vi "Actor Core.vi"(8 "error in":errorcluster, 11 "SignalProcessing in":refnum<class "SignalProcessing.lvclass">) -> (0 "error out":errorcluster, 3 "Actor out":refnum<class "Actor.lvclass">)   [LabVIEW 2019, in "SignalProcessing.lvlib" / "SignalProcessing.lvclass"]
doc: "(<B>Filename</B>: Actor Framework.lvlib:Actor.lvclass:Actor Core.vi)\n\nReceives messages to the actor, reacts to them, and initiates any error handling that may shut the actor down.\n\nDescendant classes may override this VI to append parallel tasks for the actor to complete while it handles messages. Overrides use the Call Parent Method node."
uses:
  SignalProcessing.lvclass
  C:/Program Files (x86)/National Instruments/LabVIEW 2019/vi.lib/ActorFramework/Actor/Actor.lvclass
  <vilib>/ActorFramework/Actor/Actor.lvclass
  SignalProcessing.lvclass/SignalProcessing.ctl
  <vilib>/ActorFramework/Actor/Actor.lvclass/Actor.ctl
  <vilib>/ActorFramework/Message Enqueuer/Message Enqueuer.lvclass/Message Enqueuer.ctl
  LunchTest.lvclass
  C:/Program Files (x86)/National Instruments/LabVIEW 2019/vi.lib/NI/Event Source Actor/Event Source/Event/Event.lvclass
  <vilib>/NI/Event Source Actor/Event Source/Event/Event.lvclass/Event.ctl
  <vilib>/NI/Event Source Actor/Event Source/Event Source Messages/Generate Event Msg/Generate Event Msg.lvclass/Generate Event Msg.ctl
  Exit.lvclass
  <vilib>/ActorFramework/Message Enqueuer/Init from Existing Queue.vi
  <vilib>/ActorFramework/Message Enqueuer/Enqueue.vi
  <vilib>/NI/Event Source Actor/Event Source/Event Source Messages/Generate Event Msg/Generate Event Msg.lvclass
  C:/Program Files (x86)/National Instruments/LabVIEW 2019/vi.lib/ActorFramework/Message/Message.lvclass
  SignalProcessing Global.vi
  <vilib>/ActorFramework/Message Priority Queue/Priority Enqueue.vi
  <vilib>/NI/Event Source Actor/Event Source/Event Source/Event Source.lvclass
  <vilib>/ActorFramework/Message Enqueuer/Message Enqueuer.lvclass
  <vilib>/NI/Event Source Actor/Event Source/Event/Event.lvclass
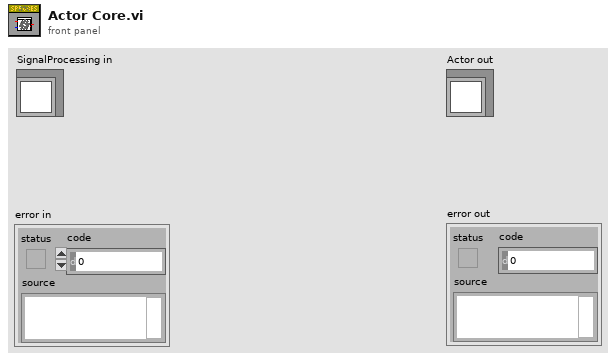
[diagram p1: front panel]
types:
  T1 = enum32{"Invalid", "Standard", "Closed", "Hidden", "Minimized", "Maximized"}
  T2 = enum32{"invalid app kind", "Development System", "Run Time System", "Student Edition", "Embedded LabVIEW", "Evaluation", "Custom"}
  T3 = cluster{"Core":cluster{"Current VI Reference":refnum<vi>, "Close Panel on Exit?":bool}, "Your Boolean data":bool, "Your string data":string}
  T4 = cluster{"Current VI Reference":refnum<vi>, "Close Panel on Exit?":bool}
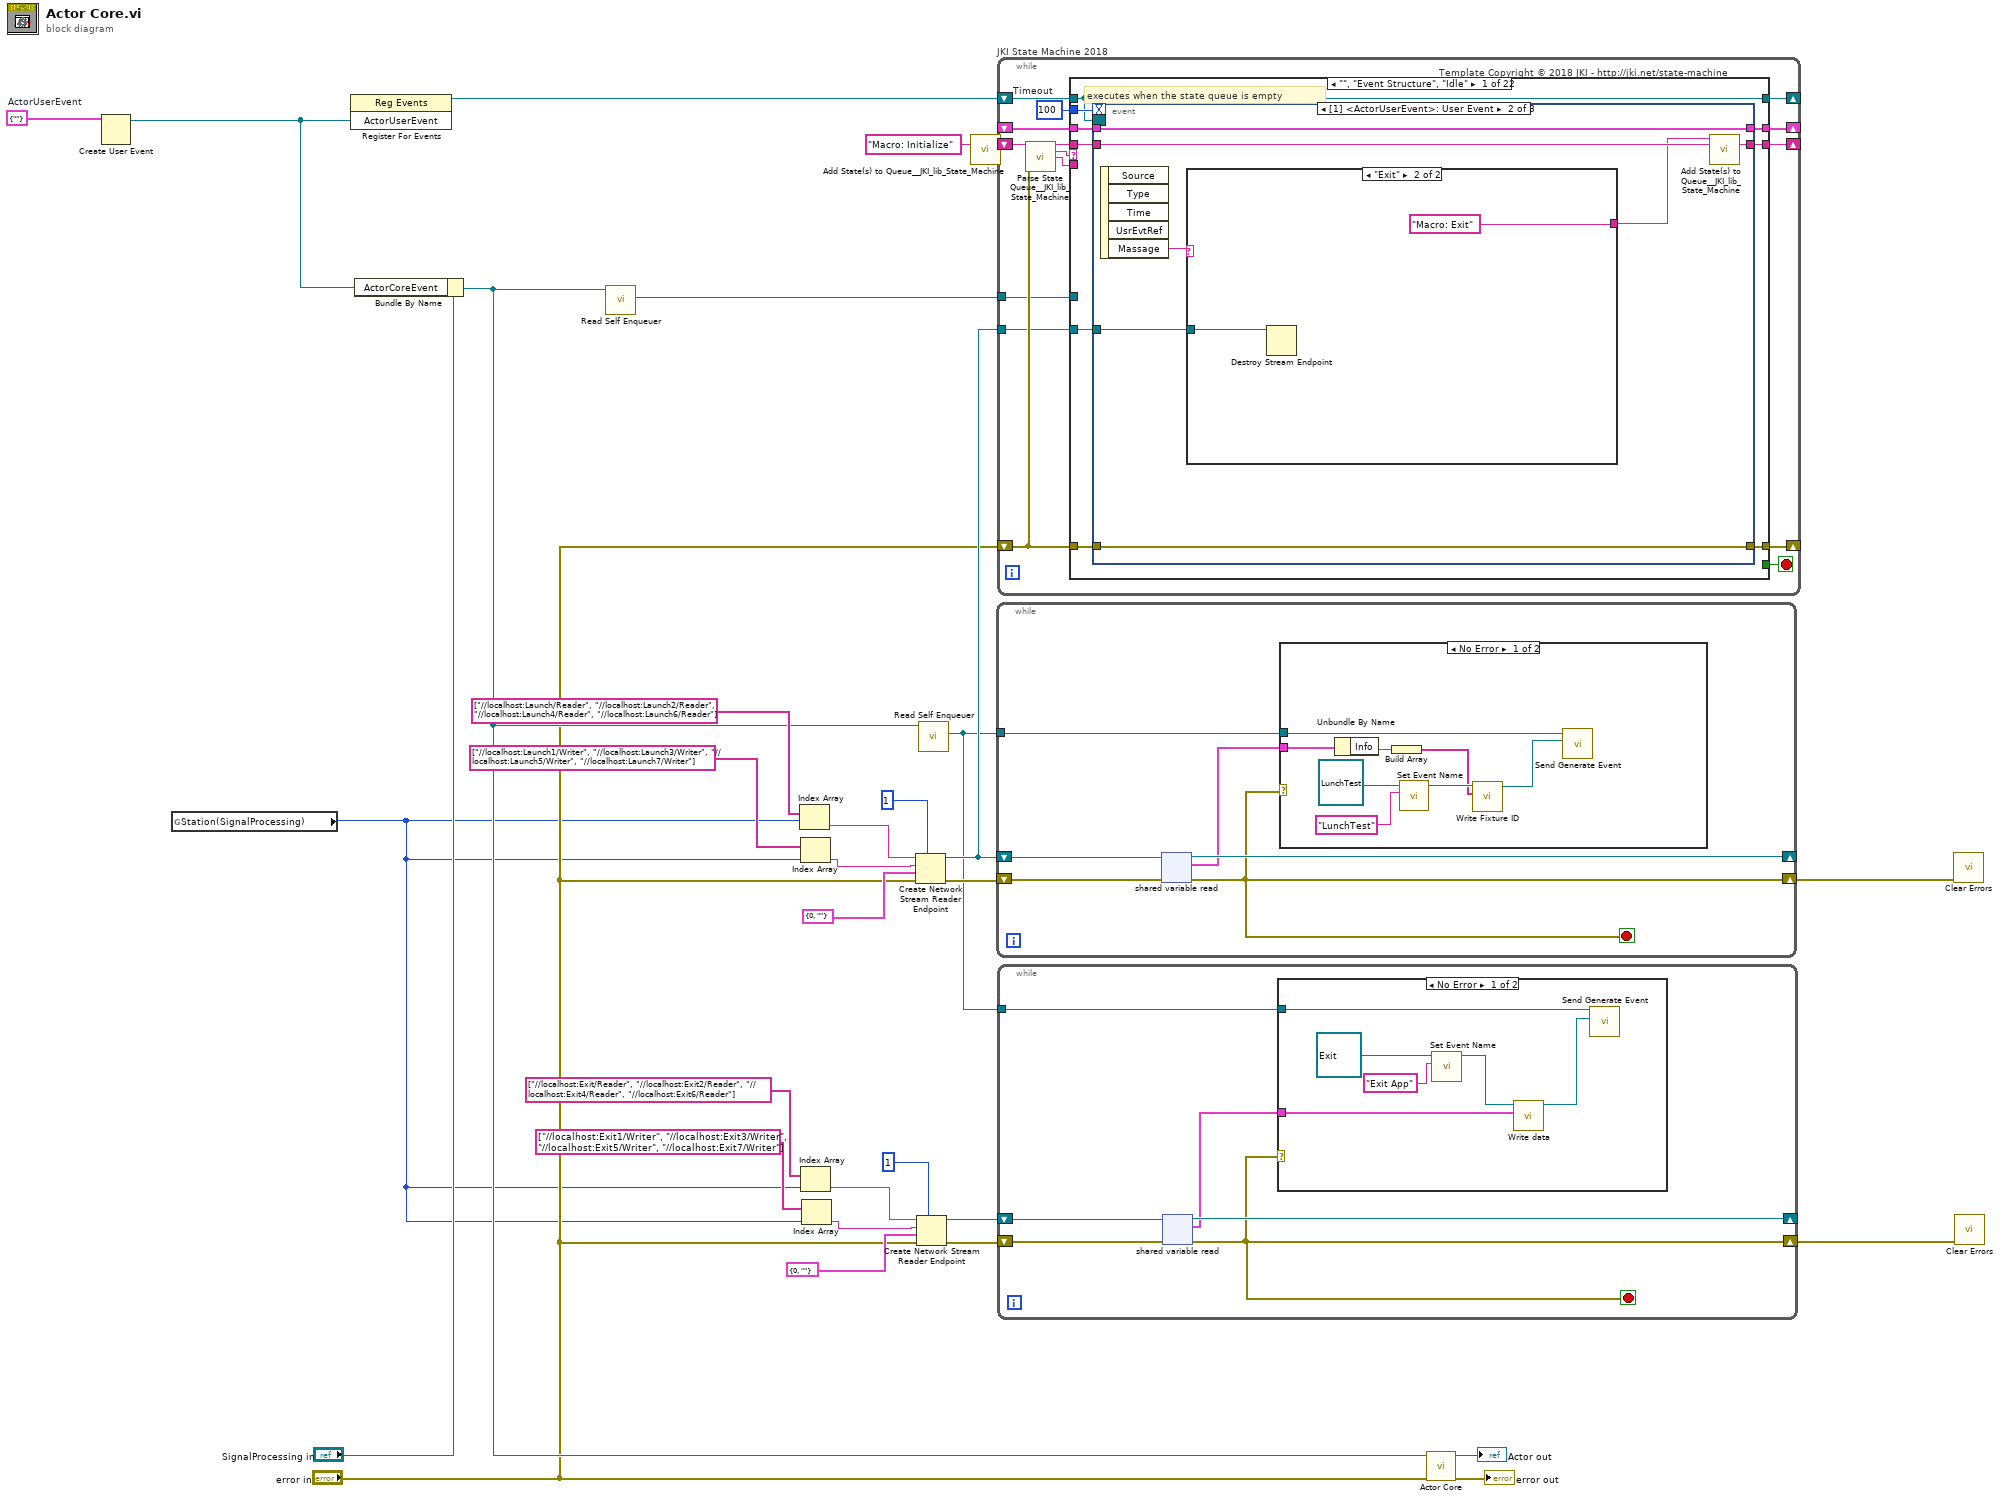
[diagram p0: block diagram]
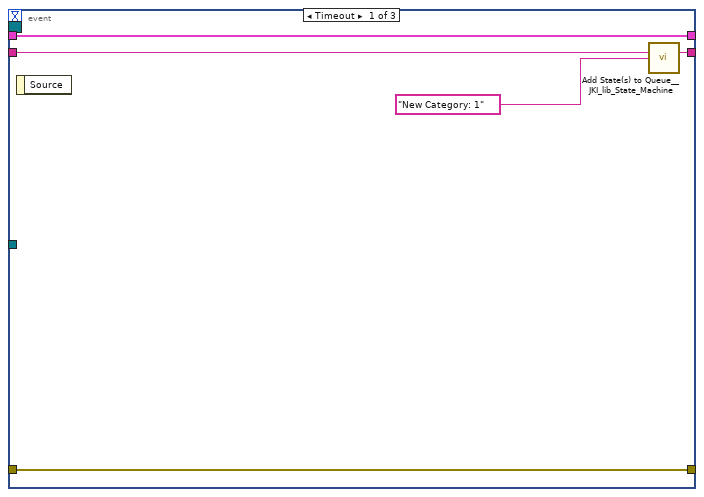
[diagram p4: hidden frame]
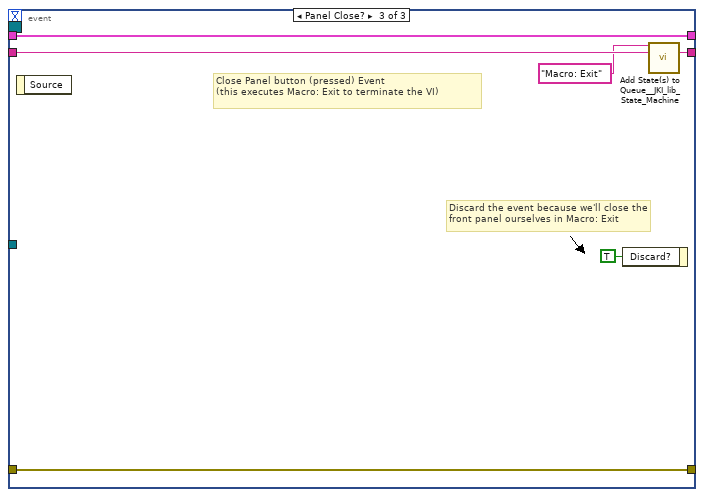
[diagram p6: hidden frame]
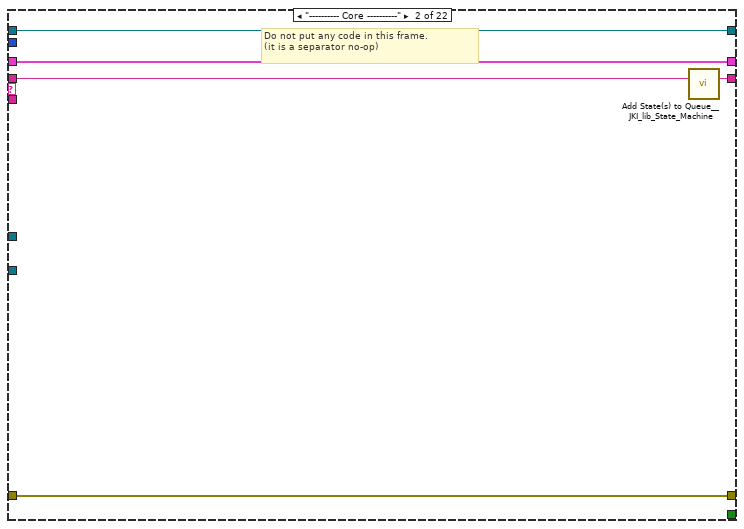
[diagram p7: hidden frame]
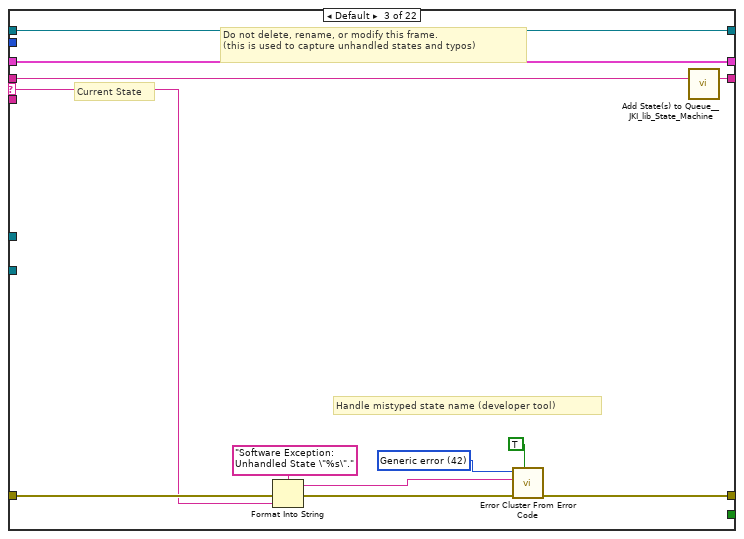
[diagram p8: hidden frame]
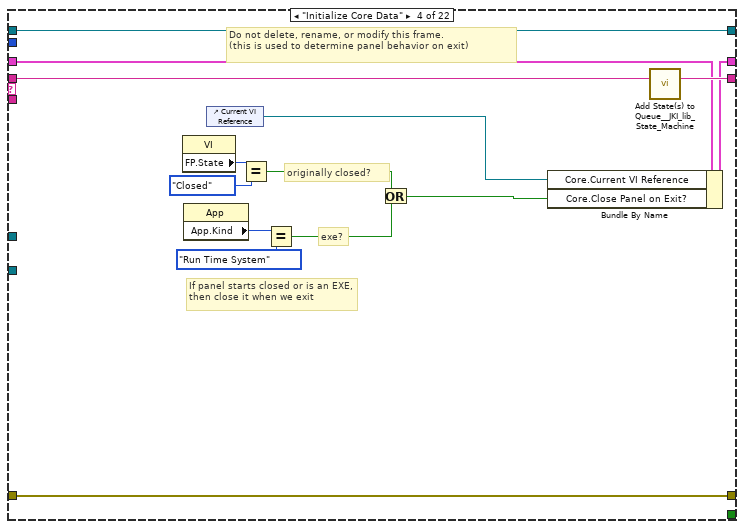
[diagram p9: hidden frame]
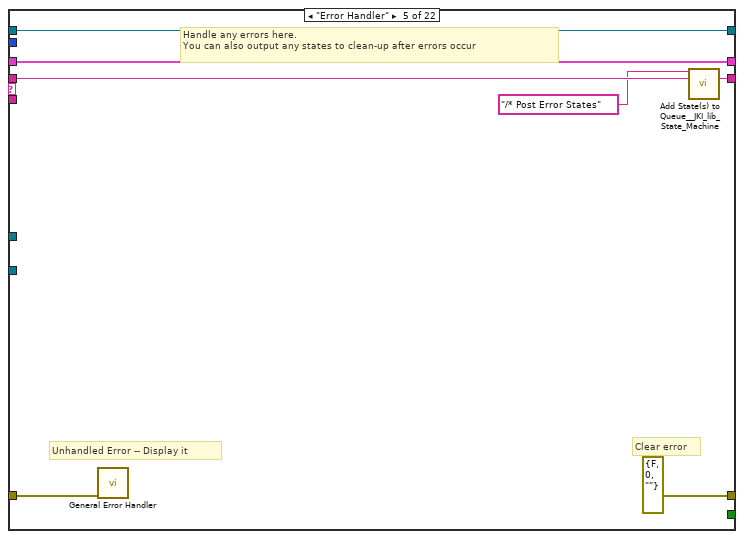
[diagram p10: hidden frame]
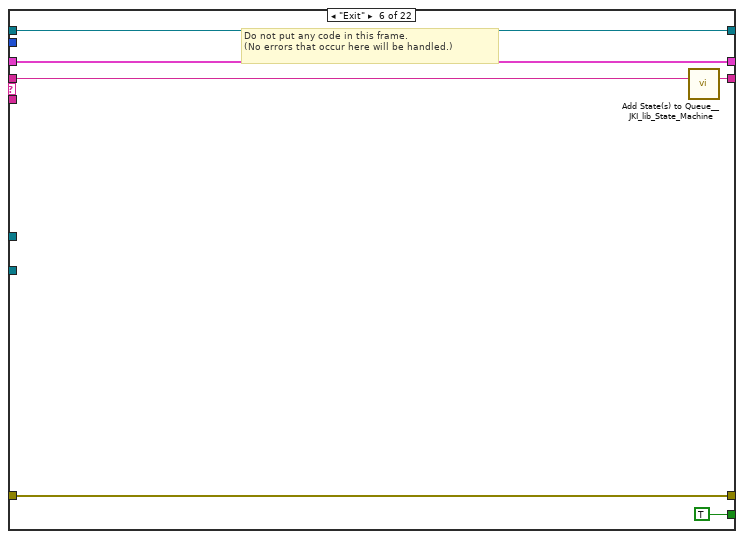
[diagram p11: hidden frame]
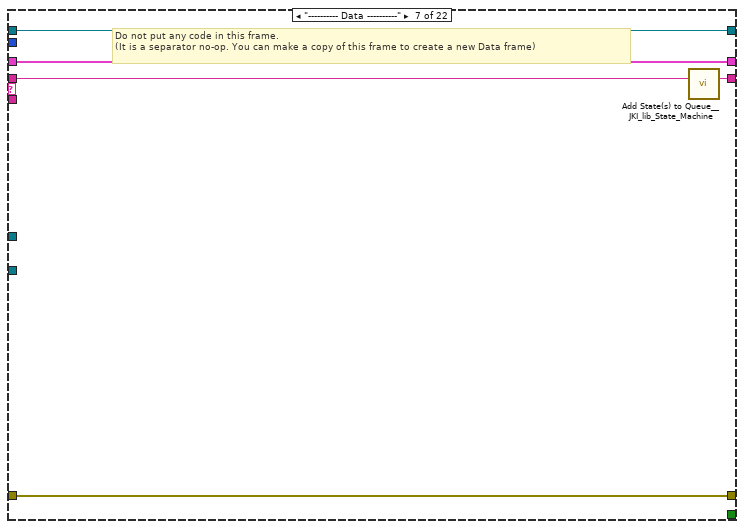
[diagram p12: hidden frame]
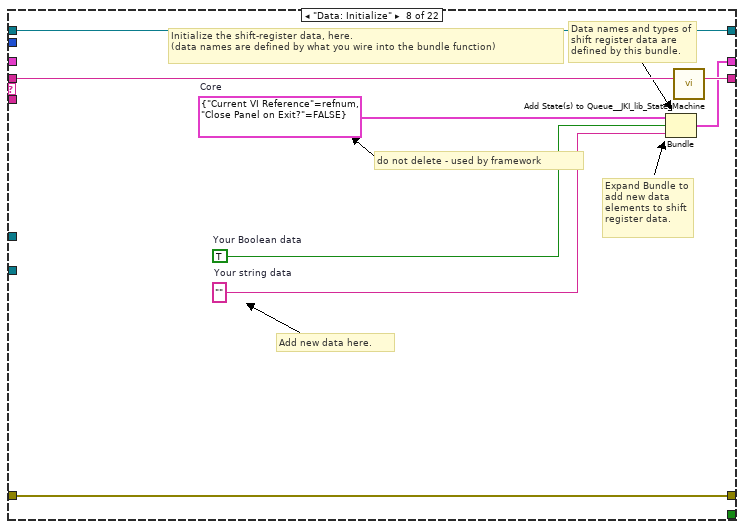
[diagram p13: hidden frame]
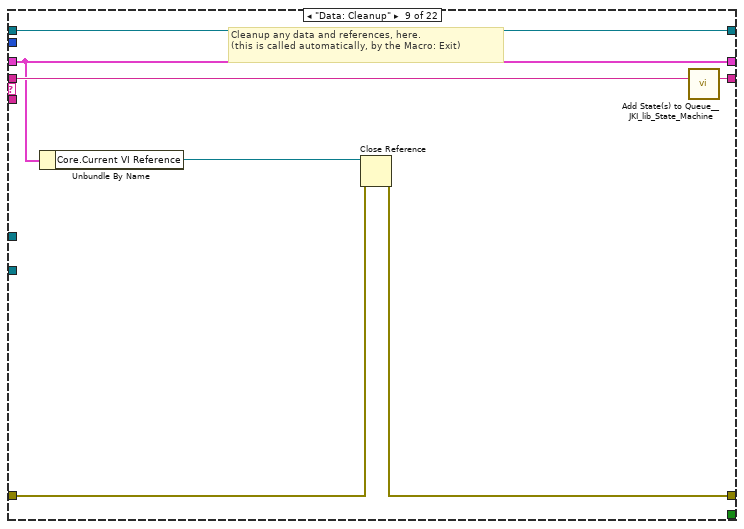
[diagram p14: hidden frame]
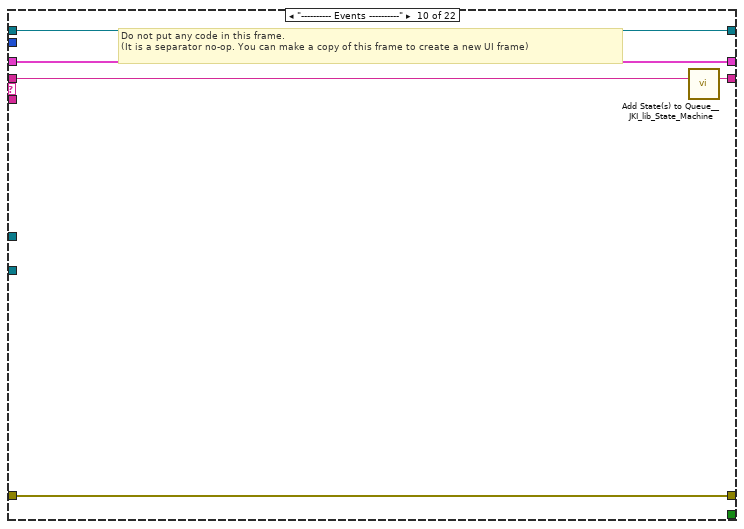
[diagram p15: hidden frame]
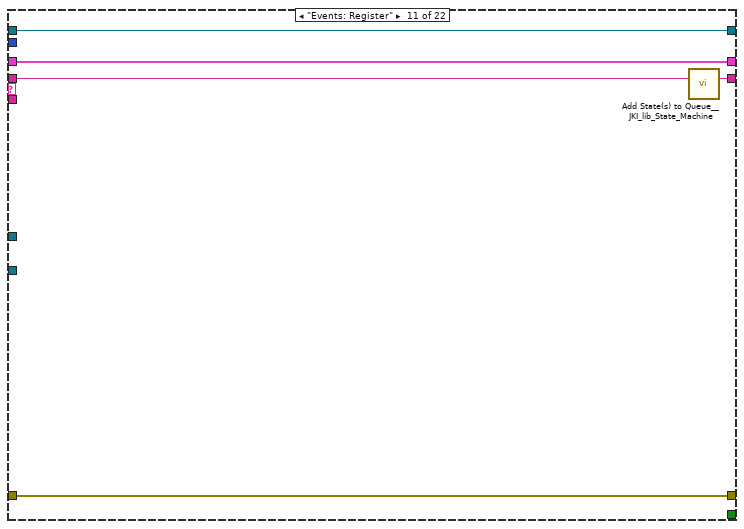
[diagram p16: hidden frame]
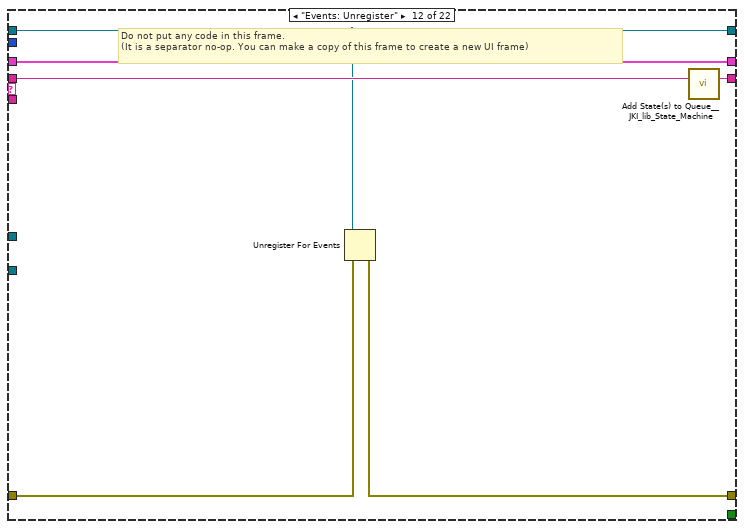
[diagram p17: hidden frame]
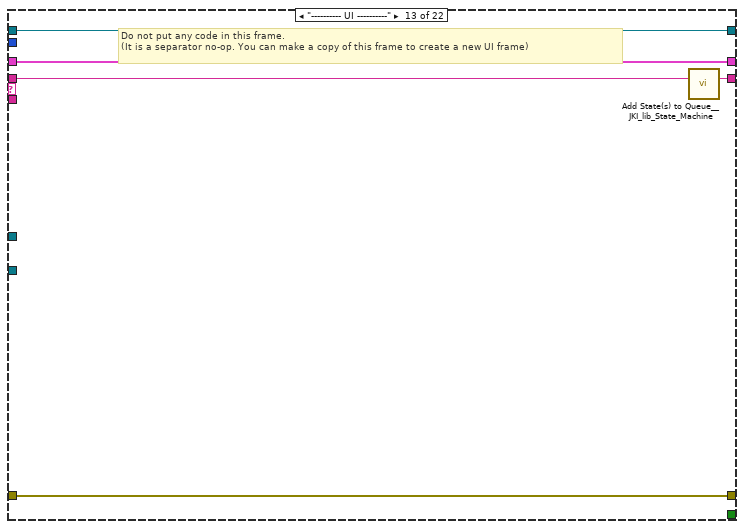
[diagram p18: hidden frame]
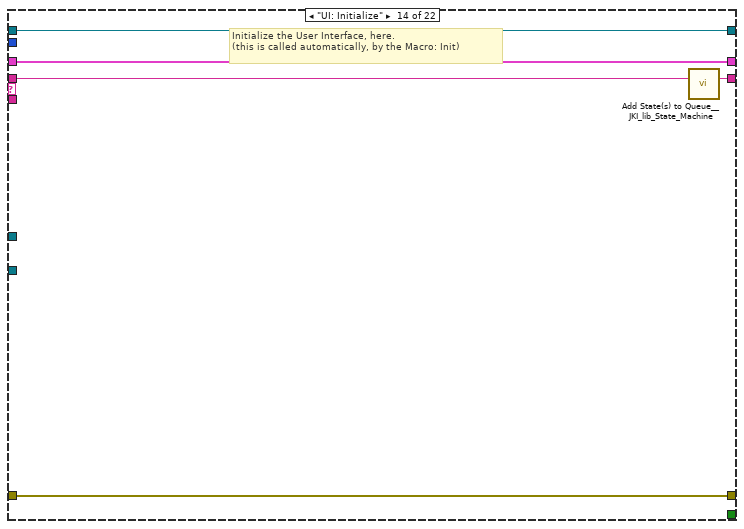
[diagram p19: hidden frame]
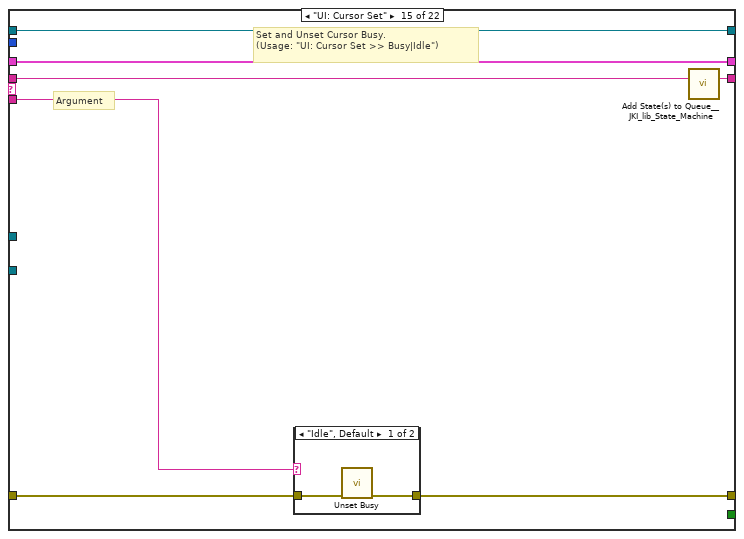
[diagram p20: hidden frame]
diagram:
  w27 = cluster{"Massage":string} {"Massage"=""}  # ActorUserEvent
  n1 = Create User Event(user event datatype=w27) -> (user event=w25:refnum<user-event>)  [unwired: 1 in, 1 out]
  n2 = global read "SignalProcessing Global.vi" "Station(SignalProcessing)"() -> (w1:i32)
  n3 = register-events(w25) -> (reference out=w26:refnum<event-registration>)  [unwired: 2 in, 1 out]
  n4 = Bundle By Name(cluster="SignalProcessing in", "ActorCoreEvent"=w25) -> (w4:refnum<class "SignalProcessing.lvclass">)
  n5 = call <vilib>:"Read Self Enqueuer.vi"("Actor"=w4) -> ("Self Enqueuer"=w24:refnum<class "Message Enqueuer.lvclass">)  [unwired: 10 in]
  n6 = Index Array(array=string[] ["//localhost:Launch/Reader", "//localhost:Launch2/Reader", "//localhost:Launch4/Reader", "//localhost:Launch6/Reader"], index=w1) -> (element=w16:string)
  n7 = Index Array(array=string[] ["//localhost:Launch1/Writer", "//localhost:Launch3/Writer", "//localhost:Launch5/Writer", "//localhost:Launch7/Writer"], index=w1) -> (element=w14:string)
  n8 = Index Array(array=string[] ["//localhost:Exit/Reader", "//localhost:Exit2/Reader", "//localhost:Exit4/Reader", "//localhost:Exit6/Reader"], index=w1) -> (element=w11:string)
  n9 = Index Array(array=string[] ["//localhost:Exit1/Writer", "//localhost:Exit3/Writer", "//localhost:Exit5/Writer", "//localhost:Exit7/Writer"], index=w1) -> (element=w13:string)
  n10 = Create Network Stream Reader Endpoint(7:1 ("reader buffer size"), 8:"error in", 9:cluster{"Socket":i32, "Info":string} {"Socket"=0, "Info"=""}, 10:w14, 11:w16) -> (0:w20:errorcluster, 3:w19:refnum<k21>)  [unwired: 2 in]
  n11 = Create Network Stream Reader Endpoint(7:1 ("reader buffer size"), 8:"error in", 9:cluster{"Socket":i32, "Info":string} {"Socket"=0, "Info"=""}, 10:w13, 11:w11) -> (0:w7:errorcluster, 3:w8:refnum<k21>)  [unwired: 2 in]
  n12 = call <vilib>:"Read Self Enqueuer.vi"("Actor"=w4) -> ("Self Enqueuer"=w2:refnum<class "Message Enqueuer.lvclass">)  [unwired: 10 in]
  n13 = call <vilib>:"Add State(s) to Queue__JKI_lib_State_Machine.vi"("State(s) in (\"\")"="Macro: Initialize") -> ("States Out"=w29:string)  [unwired: 14 in]
  n14 = while {
    tunnel: w2 -> [w32]
    shift-right: [w34] -> w18
    shift-left: w20 -> [w35]
    shift-right: [w37] -> _
    shift-left: w19 -> [w36]
    stop <- w34 stop-if-true
    n15 = shared-variable-read(w36, w35) -> (w37:refnum<k21>, w34:errorcluster, w33:cluster{"Socket":i32, "Info":string})  [unwired: 1 in, 1 out]
    n16 = case shown="No Error" w34 {
      tunnel: w33 -> [w40 _]
      tunnel: w32 -> [w42 _]
      frame No Error {
        n17 = Unbundle By Name(w40) -> ("Info"=w39:string)
        n18 = Build Array(w39) -> (w38:string[])
        n19 = call <vilib>:"Set Event Name.vi"("Name (Generic)"="LunchTest", "Event In"=refnum<class "LunchTest.lvclass"> refnum ("SignalProcessing.lvlib:LunchTest.lvclass")) -> ("Event Out"=w43:refnum<class "LunchTest.lvclass">)  [unwired: 9 in]
        n20 = call-dynamic "Write Fixture ID.vi"("Fixture ID"=w38, "LunchTest in"=w43) -> ("LunchTest out"=w41:refnum<class "LunchTest.lvclass">)  [unwired: 8 in, 1 out]
        n21 = call <vilib>:"Send Generate Event.vi"("Event"=w41, "Event Source Address"=w42) -> ()  [unwired: 8 in, 2 out]
      }
      frame Error {
      }
    }
  }
  n22 = while "JKI State Machine 2018" {
    shift-right: [w53] -> _
    shift-left: _ -> [w52]
    shift-right: [w56] -> _
    shift-left: "error in" -> [w50]
    shift-right: [w55] -> _
    shift-left: w29 -> [w57]
    shift-right: [w49] -> _
    shift-left: w26 -> [w48]
    tunnel: w24 -> [w47]
    tunnel: w19 -> [w46]
    stop <- w54 stop-if-true
    w51 = 100  # Timeout
    # "Template Copyright © 2018 JKI - http://jki.net/state-machine"
    n23 = call <vilib>:"Parse State Queue__JKI_lib_State_Machine.vi"("State Queue"=w57, "Error In (no error)"=w50) -> ("Remaining States"=w59:string, "Current State"=w60:string, "Arguments"=w58:string)  [unwired: 11 in]
    n24 = case shown="\"\", \"Event Structure\", \"Idle\"" w60 {
      selector: w60 -> [_ _ w96 _ _ _ _ _ _ _ _ _ _ _ _ _ _ _ _ _ _ _]
      tunnel: w59 -> [w69 w94 w100 w120 w127 w133 w138 w146 w153 w158 w163 w169 w174 w179 w186 w198 w268 w274 w285 w290 w295 w300]
      tunnel: w58 -> [_ _ _ _ _ _ _ _ _ _ _ _ _ _ w181 w192 _ _ _ _ _ _]
      tunnel: w52 -> [w67 w91 w98 w113 w124 w131 w135 _ w148 w155 w161 w167 w171 w177 w184 w194 w265 w271 w282 w287 w293 w297]
      tunnel: [w66 w92 w102 w117 errorcluster {"status"=FALSE, "code"=0, "source"=""} ("error out") w130 w136 w143 w149 w156 w160 w164 w172 w176 w182 w195 w266 w272 w283 w288 w291 w298] -> w56
      tunnel: w50 -> [w65 w92 w101 w117 w123 w130 w136 w143 w150 w156 w160 w165 w172 w176 w183 w196 w266 w272 w283 w288 w291 w298]
      tunnel: [w68 w93 w99 w119 w126 w132 w137 w145 w152 w157 w162 w168 w173 w178 w185 w197 w267 w273 w284 w289 w294 w299] -> w55
      tunnel: [_ _ _ _ _ TRUE _ _ _ _ _ _ _ _ _ _ _ _ _ _ _ _] -> w54
      tunnel: [w64 w91 w98 w118 w124 w131 w135 w144 w148 w155 w161 w167 w171 w177 w184 w194 w265 w271 w282 w287 w293 w297] -> w53
      tunnel: w51 -> [w63 _ _ _ _ _ _ _ _ _ _ _ _ _ _ _ _ _ _ _ _ _]
      tunnel: [w62 w90 w95 w107 w121 w128 w134 w139 w147 w154 w159 w166 w170 w175 w180 w191 w264 w269 w275 w286 w292 w296] -> w49
      tunnel: w48 -> [w62 w90 w95 w107 w121 w128 w134 w139 w147 w154 w159 w166 w170 w175 w180 w191 w264 w269 w275 w286 w292 w296]
      tunnel: w47 -> [_ _ _ _ _ _ _ _ _ _ _ _ _ _ _ _ _ _ _ _ _ _]
      tunnel: w46 -> [w61 _ _ _ _ _ _ _ _ _ _ _ _ _ _ _ _ _ _ _ _ _]
      frame "", "Event Structure", "Idle" {
        # "executes when the state queue is empty"
        n25 = event shown="[1] <ActorUserEvent>: User Event" {
          selector: w62 -> [_ _ _]
          dyn-events: _ -> [_ _ _]
          timeout: w63 -> [_ _ _]
          tunnel: w69 -> [w74 w81 w89]
          tunnel: [w73 w80 w88] -> w68
          tunnel: w67 -> [w71 w78 w86]
          tunnel: [w72 w79 w87] -> w66
          tunnel: w65 -> [w72 w79 w87]
          tunnel: [w71 w78 w86] -> w64
          tunnel: w61 -> [_ w75 _]
          event Timeout {
            n26 = event-data() -> ()  [unwired: 1 in, 1 out]
            n27 = call <vilib>:"Add State(s) to Queue__JKI_lib_State_Machine.vi"("State(s) in (\"\")"=w74, "State(s) at Back (\"\")"="New Category: 1" ("State(s) at Back (\"\")")) -> ("States Out"=w73:string)  [unwired: 13 in]
          }
          event User Event {
            n28 = event-data() -> ("Massage"=w77:string)  [unwired: 1 in, 4 out]
            n29 = case shown="\"Exit\"" w77 {
              tunnel: [_ "Macro: Exit"] -> w76
              tunnel: w75 -> [_ w82]
              frame "Idle", Default {
              }
              frame "Exit" {
                n30 = Destroy Stream Endpoint(11:w82) -> ()  [unwired: 1 in, 1 out]
              }
            }
            n31 = call <vilib>:"Add State(s) to Queue__JKI_lib_State_Machine.vi"("State(s) in Front (\"\")"=w76, "State(s) in (\"\")"=w81) -> ("States Out"=w80:string)  [unwired: 13 in]
          }
          event Panel Close? {
            # "Discard the event because we'll close the front panel ourselves in Macro: Exit"
            # "Close Panel button (pressed) Event\n(this executes Macro: Exit to terminate the VI)"
            n32 = event-data() -> ()  [unwired: 1 in, 1 out]
            n33 = event-data("Discard?"=TRUE) -> ()  [unwired: 1 in, 1 out]
            n34 = call <vilib>:"Add State(s) to Queue__JKI_lib_State_Machine.vi"("State(s) in Front (\"\")"="Macro: Exit", "State(s) in (\"\")"=w89) -> ("States Out"=w88:string)  [unwired: 13 in]
          }
        }
      }
      frame "---------- Core ----------" {
        # "Do not put any code in this frame.\n(it is a separator no-op)"
        n35 = call <vilib>:"Add State(s) to Queue__JKI_lib_State_Machine.vi"("State(s) in (\"\")"=w94) -> ("States Out"=w93:string)  [unwired: 14 in]
      }
      frame Default {
        w105 = 42 items=["No error", "Argument error", "Memory is full", "Out of zone", "End of file", "File already open", "Generic file I/O error", "File not found", "File permission error", "Disk is full", "Duplicate path", "Too many files open", "System feature not enabled", "Resource file not found", "Cannot add resource", "Resource not found", "Image not found", "Image memory error", "Pen does not exist", "Config type invalid", "Config token not found", "Config parse error", "Config memory error", "Bad external code format", "Bad external code offset", "External code not present", "Null window", "Destroy window error", "Null menu", "Print aborted", "Bad print record", "Print driver error", "Windows error during printing", "Memory error during printing", "Print dialog error", "Generic print error", "Invalid device refnum", "Device not found", "Device parameter error", "Device unit error", "Cannot open device", "Device call aborted", "Generic error", "Cancelled by user", "Object ID too low", "Object ID too high", "Object not in heap", "Unknown heap", "Unknown object (invalid DefProc)", "Unknown object (DefProc not in table)", "Message out of range", "Invalid (null) method", "Unknown message", "Manager call not supported", "Bad address", "Network operation in progress", "Network operation timed out", "Connection is busy", "Network attribute not supported", "Network error", "Address in use", "System out of memory", "Connection aborted", "Connection refused", "Not connected", "Already connected", "Connection closed", "Initialization error (interapplication manager)", "Bad occurrence", "Wait on unbound occurrence handler", "Occurrence queue overflow", "Datalog type conflict", "Unused", "Unrecognized type (interapplication manager)", "Memory corrupt", "Failed to make temporary DLL", "Old CIN version", "Drag socket not found", "Failed to load drop-object", "Failed to register OLE object", "Failed to release OLE object", "Format specifier type mismatch", "Unknown format specifier", "Too few format specifiers", "Too many format specifiers", "Scan failed", "Newer CIN version", "Error converting to variant", "Runtime menu error", "Password tampered", "Variant attribute not found", "Incompatible variant data type", "Event data is not available", "Event Store is not present", "Occurrence is not found", "Event Queue is not created", "Event info is not available", "Refnum passed is NULL", "Error retrieving Class GUID", "Error retrieving CoClass GUID", "Error retrieving TypeLib GUID.", "Bad built application magic bytes.", "Specific driver is different from the specific driver associated with the Logical Name.", "There is no session opened to the class driver.", "Max Error", "MAX - Error with config objects", "MAX - Error loading configuration", "MAX - Group not supported"]
        # "Current State"
        # "Do not delete, rename, or modify this frame.\n(this is used to capture unhandled states and typos)"
        # "Handle mistyped state name (developer tool)"
        n36 = Format Into String(format string="Software Exception: Unhandled State \"%s\"." ("message"), error in=w101, w96) -> (resulting string=w104:string, error out=w103:errorcluster)  [unwired: 1 in]
        n37 = call <vilib>:"Error Cluster From Error Code.vi"("show call chain? (False)"=TRUE, "error in (no error)"=w103, "error message (\"\")"=w104, "error code (0)"=w105) -> ("error out"=w102:errorcluster)  [unwired: 5 in]
        n38 = call <vilib>:"Add State(s) to Queue__JKI_lib_State_Machine.vi"("State(s) in (\"\")"=w100) -> ("States Out"=w99:string)  [unwired: 14 in]
      }
      frame "Initialize Core Data" {
        # "Do not delete, rename, or modify this frame.\n(this is used to determine panel behavior on exit)"
        # "originally closed?"
        # "exe?"
        # "If panel starts closed or is an EXE, then close it when we exit"
        n39 = property class="VI"() -> ("FP.State"=w110:T1)  [unwired: 2 in, 2 out]
        n40 = property class="App"() -> ("App.Kind"=w116:T2)  [unwired: 2 in, 2 out]
        n41 = control-ref of="Current VI Reference"() -> (w111:refnum<vi>)
        n42 = Equal?(x=w110, y=T1."Closed" ("Front Panel Window:State")) -> (x = y?=w108:bool)
        n43 = Equal?(x=w116, y=T2."Run Time System" ("Application:Kind")) -> (x = y?=w114:bool)
        n44 = Or(x=w108, y=w114) -> (x .or. y?=w112:bool)
        n45 = Bundle By Name(cluster=w113, "Core.Current VI Reference"=w111, "Core.Close Panel on Exit?"=w112) -> (w118:T3)
        n46 = call <vilib>:"Add State(s) to Queue__JKI_lib_State_Machine.vi"("State(s) in (\"\")"=w120) -> ("States Out"=w119:string)  [unwired: 14 in]
      }
      frame "Error Handler" {
        # "Unhandled Error -- Display it"
        # "Handle any errors here.\nYou can also output any states to clean-up after errors occur"
        # "Clear error"
        n47 = call <vilib>:"General Error Handler.vi"("error in (no error)"=w123) -> ()  [unwired: 10 in, 5 out]
        n48 = call <vilib>:"Add State(s) to Queue__JKI_lib_State_Machine.vi"("State(s) in Front (\"\")"="/* Post Error States", "State(s) in (\"\")"=w127) -> ("States Out"=w126:string)  [unwired: 13 in]
      }
      frame "Exit" {
        # "Do not put any code in this frame.\n(No errors that occur here will be handled.)"
        n49 = call <vilib>:"Add State(s) to Queue__JKI_lib_State_Machine.vi"("State(s) in (\"\")"=w133) -> ("States Out"=w132:string)  [unwired: 14 in]
      }
      frame "---------- Data ----------" {
        # "Do not put any code in this frame.\n(It is a separator no-op. You can make a copy of this frame to create a new Data frame)"
        n50 = call <vilib>:"Add State(s) to Queue__JKI_lib_State_Machine.vi"("State(s) in (\"\")"=w138) -> ("States Out"=w137:string)  [unwired: 14 in]
      }
      frame "Data: Initialize" {
        w140 = T4 {"Current VI Reference"=refnum, "Close Panel on Exit?"=FALSE}  # Core
        w142 = TRUE  # Your Boolean data
        w141 = ""  # Your string data
        # "do not delete - used by framework"
        # "Expand Bundle to add new data elements to shift register data."
        # "Add new data here."
        # "Data names and types of shift register data are defined by this bundle."
        # "Initialize the shift-register data, here.\n(data names are defined by what you wire into the bundle function)"
        n51 = Bundle("Core"=w140, "Your Boolean data"=w142, "Your string data"=w141) -> (w144:T3)  [unwired: 1 in]
        n52 = call <vilib>:"Add State(s) to Queue__JKI_lib_State_Machine.vi"("State(s) in (\"\")"=w146) -> ("States Out"=w145:string)  [unwired: 14 in]
      }
      frame "Data: Cleanup" {
        # "Cleanup any data and references, here.\n(this is called automatically, by the Macro: Exit)"
        n53 = Unbundle By Name(w148) -> ("Core.Current VI Reference"=w151:refnum<vi>)
        n54 = Close Reference(reference=w151, error in (no error)=w150) -> (error out=w149:errorcluster)
        n55 = call <vilib>:"Add State(s) to Queue__JKI_lib_State_Machine.vi"("State(s) in (\"\")"=w153) -> ("States Out"=w152:string)  [unwired: 14 in]
      }
      frame "---------- Events ----------" {
        # "Do not put any code in this frame.\n(It is a separator no-op. You can make a copy of this frame to create a new UI frame)"
        n56 = call <vilib>:"Add State(s) to Queue__JKI_lib_State_Machine.vi"("State(s) in (\"\")"=w158) -> ("States Out"=w157:string)  [unwired: 14 in]
      }
      frame "Events: Register" {
        n57 = call <vilib>:"Add State(s) to Queue__JKI_lib_State_Machine.vi"("State(s) in (\"\")"=w163) -> ("States Out"=w162:string)  [unwired: 14 in]
      }
      frame "Events: Unregister" {
        # "Do not put any code in this frame.\n(It is a separator no-op. You can make a copy of this frame to create a new UI frame)"
        n58 = Unregister For Events(event registration refnum=w166, error in=w165) -> (error out=w164:errorcluster)
        n59 = call <vilib>:"Add State(s) to Queue__JKI_lib_State_Machine.vi"("State(s) in (\"\")"=w169) -> ("States Out"=w168:string)  [unwired: 14 in]
      }
      frame "---------- UI ----------" {
        # "Do not put any code in this frame.\n(It is a separator no-op. You can make a copy of this frame to create a new UI frame)"
        n60 = call <vilib>:"Add State(s) to Queue__JKI_lib_State_Machine.vi"("State(s) in (\"\")"=w174) -> ("States Out"=w173:string)  [unwired: 14 in]
      }
      frame "UI: Initialize" {
        # "Initialize the User Interface, here.\n(this is called automatically, by the Macro: Init)"
        n61 = call <vilib>:"Add State(s) to Queue__JKI_lib_State_Machine.vi"("State(s) in (\"\")"=w179) -> ("States Out"=w178:string)  [unwired: 14 in]
      }
      frame "UI: Cursor Set" {
        # "Argument"
        # "Set and Unset Cursor Busy.\n(Usage: \"UI: Cursor Set >> Busy|Idle\")"
        n62 = case shown="\"Idle\", Default" w181 {
          tunnel: w183 -> [w188 w190]
          tunnel: [w187 w189] -> w182
          frame "Idle", Default {
            n63 = call <vilib>:"Unset Busy.vi"("error in (no error)"=w188) -> ("error out"=w187:errorcluster)  [unwired: 10 in]
          }
          frame "Busy" {
            n64 = call <vilib>:"Set Busy.vi"("error in (no error)"=w190) -> ("error out"=w189:errorcluster)  [unwired: 9 in, 1 out]
          }
        }
        n65 = call <vilib>:"Add State(s) to Queue__JKI_lib_State_Machine.vi"("State(s) in (\"\")"=w186) -> ("States Out"=w185:string)  [unwired: 14 in]
      }
      frame "UI: Front Panel State" {
        # "Argument"
        # "Set Front Panel Open or Closed\n(Usage: \"UI: Front Panel State >> Open|Close\")"
        n66 = Unbundle By Name(w194) -> ("Core.Current VI Reference"=w193:refnum<vi>)
        n67 = case shown="\"Minimize\", \"Minimized\"" w192 {
          tunnel: w196 -> [w204 w219 w230 w243 w256]
          tunnel: [w206 w220 w232 w245 w258] -> w195
          tunnel: w193 -> [w205 w217 w231 w244 w257]
          frame "Open", "Standard", Default {
            w199 = T1."Standard" ("State")
            n68 = property class="VI"(reference=w205, error in=w204) -> (reference out=w202:refnum<vi>, error out=w203:errorcluster, "FP.State"=w201:T1)
            n69 = Not Equal?(x=w201, y=w199) -> (x != y?=w200:bool)
            n70 = case shown="True" w200 {
              tunnel: [w210 w212] -> w206
              tunnel: w203 -> [w209 w212]
              tunnel: w202 -> [w208 _]
              tunnel: w199 -> [w207 _]
              frame True {
                n71 = invoke class="VI" method="FP.Open"(reference=w208, error in=w209, "Activate"=TRUE, "State"=w207) -> (error out=w210:errorcluster)  [unwired: 1 in, 4 out]
              }
              frame False {
              }
            }
          }
          frame "Close", "Closed" {
            n72 = property class="VI"(reference=w217, error in=w219) -> (reference out=w216:refnum<vi>, error out=w218:errorcluster, "FP.State"=w214:T1)
            n73 = Not Equal?(x=w214, y=T1."Closed" ("Front Panel Window:State")) -> (x != y?=w213:bool)
            n74 = case shown="True" w213 {
              tunnel: [w221 w224] -> w220
              tunnel: w218 -> [w221 w223]
              tunnel: w216 -> [_ w222]
              frame False {
              }
              frame True {
                n75 = invoke class="VI" method="FP.Close"(reference=w222, error in=w223) -> (error out=w224:errorcluster)  [unwired: 1 in, 2 out]
              }
            }
          }
          frame "Hidden", "Hide" {
            w225 = T1."Hidden" ("State")
            n76 = property class="VI"(reference=w231, error in=w230) -> (reference out=w228:refnum<vi>, error out=w229:errorcluster, "FP.State"=w227:T1)
            n77 = Not Equal?(x=w227, y=w225) -> (x != y?=w226:bool)
            n78 = case shown="True" w226 {
              tunnel: [w236 w237] -> w232
              tunnel: w229 -> [w235 w237]
              tunnel: w228 -> [w234 _]
              tunnel: w225 -> [w233 _]
              frame True {
                n79 = invoke class="VI" method="FP.Open"(reference=w234, error in=w235, "State"=w233) -> (error out=w236:errorcluster)  [unwired: 2 in, 4 out]
              }
              frame False {
              }
            }
          }
          frame "Minimize", "Minimized" {
            w238 = T1."Minimized" ("State")
            n80 = property class="VI"(reference=w244, error in=w243) -> (reference out=w241:refnum<vi>, error out=w242:errorcluster, "FP.State"=w240:T1)
            n81 = Not Equal?(x=w240, y=w238) -> (x != y?=w239:bool)
            n82 = case shown="True" w239 {
              tunnel: [w249 w250] -> w245
              tunnel: w242 -> [w248 w250]
              tunnel: w241 -> [w247 _]
              tunnel: w238 -> [w246 _]
              frame True {
                n83 = invoke class="VI" method="FP.Open"(reference=w247, error in=w248, "State"=w246) -> (error out=w249:errorcluster)  [unwired: 2 in, 4 out]
              }
              frame False {
              }
            }
          }
          frame "Maximize", "Maximized" {
            w251 = T1."Maximized" ("State")
            n84 = property class="VI"(reference=w257, error in=w256) -> (reference out=w254:refnum<vi>, error out=w255:errorcluster, "FP.State"=w253:T1)
            n85 = Not Equal?(x=w253, y=w251) -> (x != y?=w252:bool)
            n86 = case shown="True" w252 {
              tunnel: [w262 w263] -> w258
              tunnel: w255 -> [w261 w263]
              tunnel: w254 -> [w260 _]
              tunnel: w251 -> [w259 _]
              frame True {
                n87 = invoke class="VI" method="FP.Open"(reference=w260, error in=w261, "State"=w259) -> (error out=w262:errorcluster)  [unwired: 2 in, 4 out]
              }
              frame False {
              }
            }
          }
        }
        n88 = call <vilib>:"Add State(s) to Queue__JKI_lib_State_Machine.vi"("State(s) in (\"\")"=w198) -> ("States Out"=w197:string)  [unwired: 14 in]
      }
      frame "---------- Macro ----------" {
        # "Do not put any code in this frame.\n(It is a separator no-op. You can make a copy of this frame to create a new Macro frame)"
        n89 = call <vilib>:"Add State(s) to Queue__JKI_lib_State_Machine.vi"("State(s) in (\"\")"=w268) -> ("States Out"=w267:string)  [unwired: 14 in]
      }
      frame "Macro: Initialize" {
        # "Initialization Macro\n(This is called once, when the VI starts)"
        n90 = call <vilib>:"Add State(s) to Queue__JKI_lib_State_Machine.vi"("State(s) in Front (\"\")"="Data: Initialize\nInitialize Core Data\nEvents: Register\nUI: Initialize\nUI: Front Panel State >> Close", "State(s) in (\"\")"=w274) -> ("States Out"=w273:string)  [unwired: 13 in]
      }
      frame "Macro: Exit" {
        # "Exit Macro\n(This is called once, when the VI exits)"
        n91 = Unbundle By Name(w282) -> ("Core.Close Panel on Exit?"=w281:bool)
        n92 = Select(t="UI: Front Panel State >> Close", s=w281, f="") -> (s? t:f=w278:string)
        n93 = call <vilib>:"Add State(s) to Queue__JKI_lib_State_Machine.vi"("State(s) in (\"\")"=w278, "State(s) at Back (\"\")"="Data: Cleanup\nEvents: Unregister\nExit") -> ("States Out"=w276:string)  [unwired: 13 in]
        n94 = call <vilib>:"Add State(s) to Queue__JKI_lib_State_Machine.vi"("State(s) in Front (\"\")"=w276, "State(s) in (\"\")"=w285) -> ("States Out"=w284:string)  [unwired: 13 in]
      }
      frame "---------- New Category ----------" {
        # "Template Separator\n(You can make a copy of, or modify, this frame)"
        n95 = call <vilib>:"Add State(s) to Queue__JKI_lib_State_Machine.vi"("State(s) in (\"\")"=w290) -> ("States Out"=w289:string)  [unwired: 14 in]
      }
      frame "New Category: 1" {
        n96 = call <vilib>:"Add State(s) to Queue__JKI_lib_State_Machine.vi"("State(s) in (\"\")"=w295) -> ("States Out"=w294:string)  [unwired: 14 in]
      }
      frame "New Category: 2" {
        # "Your code here.\n(You can make a copy of, or modify, this frame)"
        n97 = call <vilib>:"Add State(s) to Queue__JKI_lib_State_Machine.vi"("State(s) in (\"\")"=w300) -> ("States Out"=w299:string)  [unwired: 14 in]
      }
    }
  }
  n98 = while {
    shift-right: [w303] -> w9
    shift-left: w7 -> [w304]
    shift-right: [w306] -> _
    shift-left: w8 -> [w305]
    tunnel: w2 -> [w301]
    stop <- w303 stop-if-true
    n99 = shared-variable-read(w305, w304) -> (w306:refnum<k21>, w303:errorcluster, w302:cluster{"Socket":i32, "Info":string})  [unwired: 1 in, 1 out]
    n100 = case shown="No Error" w303 {
      tunnel: w302 -> [w309 _]
      tunnel: w301 -> [w308 _]
      frame No Error {
        n101 = call <vilib>:"Set Event Name.vi"("Name (Generic)"="Exit App", "Event In"=refnum<class "Exit.lvclass"> refnum ("SignalProcessing.lvlib:Exit.lvclass")) -> ("Event Out"=w310:refnum<class "Exit.lvclass">)  [unwired: 9 in]
        n102 = call-dynamic "Write data.vi"("data"=w309, "Exit in"=w310) -> ("Exit out"=w307:refnum<class "Exit.lvclass">)  [unwired: 8 in, 1 out]
        n103 = call <vilib>:"Send Generate Event.vi"("Event"=w307, "Event Source Address"=w308) -> ()  [unwired: 8 in, 2 out]
      }
      frame Error {
      }
    }
  }
  n104 = call-parent "Actor Core.vi"("error in"="error in", "Actor in"=w4) -> ("error out"=→"error out":errorcluster, "Actor out"=→"Actor out":refnum<class "Actor.lvclass">)  [unwired: 8 in]
  n105 = call <vilib>:"Clear Errors.vi"("error in (no error)"=w18) -> ()  [unwired: 5 in, 2 out]
  n106 = call <vilib>:"Clear Errors.vi"("error in (no error)"=w9) -> ()  [unwired: 5 in, 2 out]
